vi "Header Footer Modify Image Cell.vi"(2 "Header or Footer":T1, 5 "Modify Image Cell":bool, 9 "Header or Footer Complete Cluster IN":T2, 11 "error in (no error)":errorcluster) -> (10 "Header or Footer Complete Cluster OUT":T2, 15 "error out":errorcluster)   [LabVIEW 2013]
doc: "Version 1.0\nDeveloped by Jean-Marc Simard\nCopyright © 2010, Exaprom Inc.\nAll rights reserved.\nLicense: BSD\n\nWith iTextSharp 4.1.6 (http://itextsharp.sourceforge.net)\nunder Mozilla Public License Version 1.1\n(http://www.mozilla.org/MPL/MPL-1.1.html)"
uses:
  Controls/Header Footer Complete Cluster.ctl
  Controls/Header Footer Cluster with references.ctl
  Controls/Header Footer Type.ctl
  Controls/Header footer horiz alignment.ctl
  Controls/Cell Vertical alignment.ctl
  Controls/Page number.ctl
  C:/Users/MaxCorp/Documents/GitHub/TopView/DLL/itextsharp.dll
  DLL/itextsharp.dll
  Controls/Font cluster.ctl
  Controls/Font size.ctl
  Controls/Font color.ctl
  Controls/Header Footer Line.ctl
  Controls/Header or Footer.ctl
panel:
  # "X"
  # "Y"
  # "X"
  # "Y"
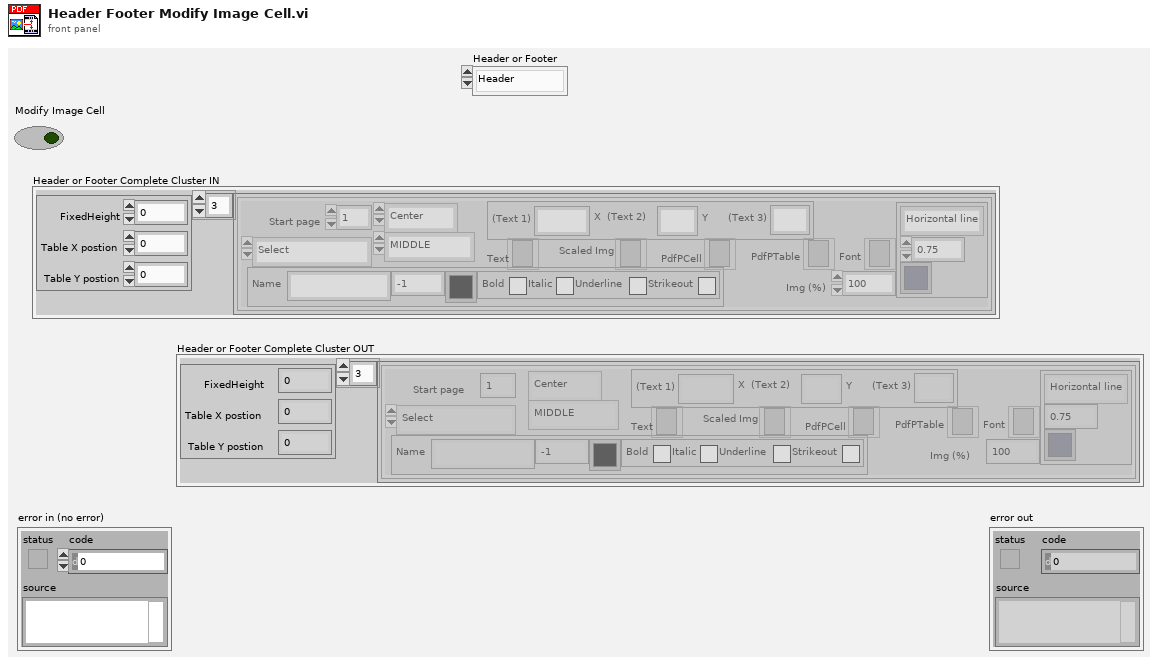
[diagram p1: front panel]
types:
  T1 = typedef "Header or Footer.ctl" = enum16{"Header", "Footer"}
  T2 = typedef "Header Footer Complete Cluster.ctl" = cluster{"Table position":cluster{"FixedHeight":dbl, "Table X postion":dbl, "Table Y postion":dbl}, "Header Footer Cluster with references [ ]":T3[]}
  T3 = typedef "Header Footer Cluster with references.ctl" = cluster{"Start page":i32, "Type":T4, "Alignment":T5, "Vertical Alignement":T6, "Page #":T7, "Text":refnum<k24>, "Scaled Img":refnum<k24>, "PdfPCell":refnum<k24>, "PdfPTable":refnum<k24>, "Font Cluster":T8, "Font ":refnum<k24>, "Img (%)":sgl, "Line":cluster{"Line":T11, "Thickness (points)":sgl, "Colour":T10}}
  T4 = typedef "Header Footer Type.ctl" = enum16{"Select", "Text", "Text + hyperlink", "Page number", "Image", "Image + hyperlink"}
  T5 = typedef "Header footer horiz alignment.ctl" = enum16{"Left", "Center", "Right"}
  T6 = typedef "Cell Vertical alignment.ctl" = enum16{"TOP", "MIDDLE", "BOTTOM"}
  T7 = typedef "Page number.ctl" = cluster{"Text 1":string, "Text 2":string, "Text 3":string}
  T8 = typedef "Font cluster.ctl" = cluster{"Name":string, "Size":T9, "Color":T10, "Style":cluster{"Bold":bool, "Italic":bool, "Underline":bool, "Strikeout":bool}}
  T9 = typedef "Font size.ctl" = sgl
  T10 = typedef "Font color.ctl" = u32
  T11 = typedef "Header Footer Line.ctl" = enum16{"No line", "Horizontal line"}
  T12 = cluster{"FixedHeight":dbl, "Table X postion":dbl, "Table Y postion":dbl}
  T13 = cluster{"Table position":cluster{"FixedHeight":dbl, "Table X postion":dbl, "Table Y postion":dbl}, "Header Footer Cluster with references [ ]":T3[]}
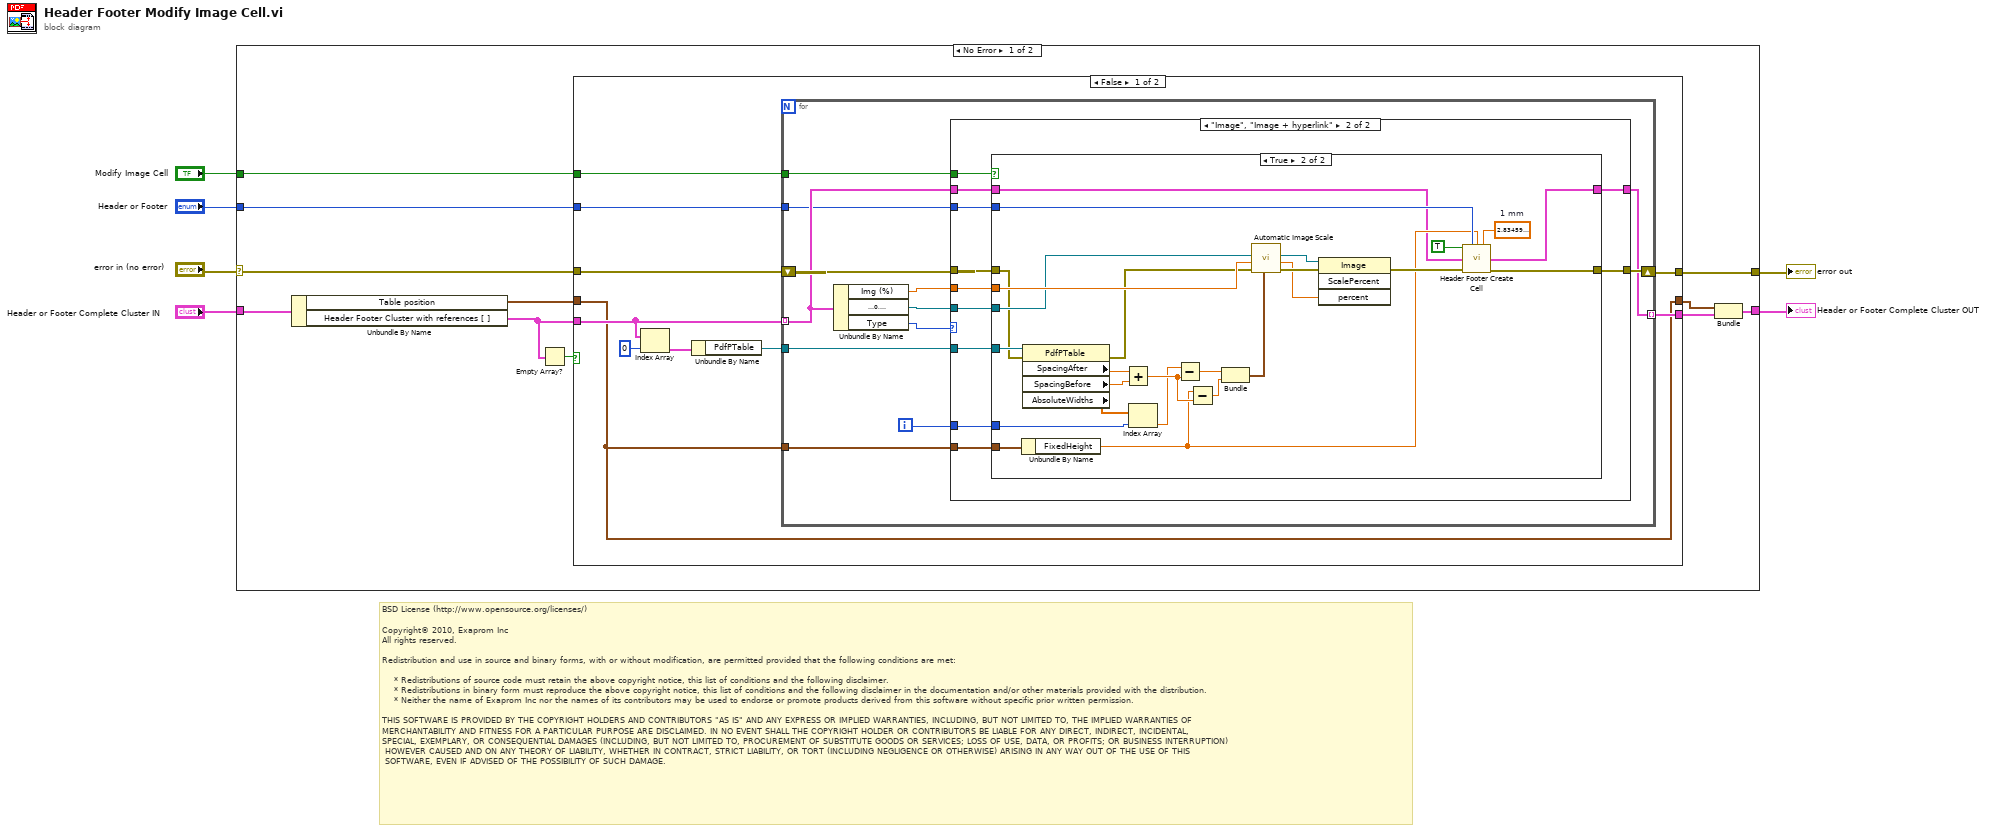
[diagram p0: block diagram]
diagram:
  # "BSD License (http://www.opensource.org/licenses/)\n\nCopyright© 2010, Exaprom Inc\nAll rights reserved.\n\nRedistribution and use in source and binary forms, with or without modification, are permitted provided that the following conditions are met:\n\n    * Redistributions of source code must retain the above copyright notice, this list of conditions and the following disclaimer.\n    * Redistributions in binary form must reproduce the above copyright notice, this list of conditions and the following disclaimer in the documentation and/or other materials provided with the distribution.\n    * Neither the name of Exaprom Inc nor the names of its contributors may be used to endorse or promote products derived from this software without specific prior written permission.\n\nTHIS SOFTWARE IS PROVIDED BY THE COPYRIGHT HOLDERS AND CONTRIBUTORS \"AS IS\" AND ANY EXPRESS OR IMPLIED WARRANTIES, INCLUDING, BUT NOT LIMITED TO, THE IMPLIED WARRANTIES OF \nMERCHANTABILITY AND FITNESS FOR A PARTICULAR PURPOSE ARE DISCLAIMED. IN NO EVENT SHALL THE COPYRIGHT HOLDER OR CONTRIBUTORS BE LIABLE FOR ANY DIRECT, INDIRECT, INCIDENTAL,\nSPECIAL, EXEMPLARY, OR CONSEQUENTIAL DAMAGES (INCLUDING, BUT NOT LIMITED TO, PROCUREMENT OF SUBSTITUTE GOODS OR SERVICES; LOSS OF USE, DATA, OR PROFITS; OR BUSINESS INTERRUPTION)\n HOWEVER CAUSED AND ON ANY THEORY OF LIABILITY, WHETHER IN CONTRACT, STRICT LIABILITY, OR TORT (INCLUDING NEGLIGENCE OR OTHERWISE) ARISING IN ANY WAY OUT OF THE USE OF THIS\n SOFTWARE, EVEN IF ADVISED OF THE POSSIBILITY OF SUCH DAMAGE."
  n1 = case shown="No Error" "error in (no error)" {
    selector: "error in (no error)" -> [w16 w85]
    tunnel: "Header or Footer Complete Cluster IN" -> [w15 w84]
    tunnel: [w17 w85] -> w6
    tunnel: [w14 w84] -> w2
    tunnel: "Header or Footer" -> [w13 _]
    tunnel: "Modify Image Cell" -> [w10 _]
    frame No Error {
      n2 = Unbundle By Name(w15) -> ("Table position"=w11:T12, "Header Footer Cluster with references [ ]"=w7:T3[])
      n3 = Empty Array?(array=w7) -> (empty?=w8:bool)
      n4 = case shown="False" w8 {
        tunnel: [w27 w83] -> w17
        tunnel: w16 -> [w26 w83]
        tunnel: w7 -> [w22 w82]
        tunnel: w13 -> [w21 _]
        tunnel: [w20 w82] -> w12
        tunnel: w11 -> [w18 w81]
        tunnel: w10 -> [w19 _]
        tunnel: [w18 w81] -> w9
        frame False {
          n5 = Index Array(array=w22, index=0) -> (element=w24:T3)
          n6 = Unbundle By Name(w24) -> ("PdfPTable"=w23:refnum<k24>)
          n7 = for {
            tunnel: w22 -> [w32] mode=indexing
            tunnel: w23 -> [w35]
            tunnel: w18 -> [w37]
            shift-right: [w30] -> w27
            shift-left: w26 -> [w38]
            tunnel: w21 -> [w31]
            tunnel: [w29] -> w20 mode=indexing
            tunnel: w19 -> [w28]
            i -> [w36]
            n8 = Unbundle By Name(w32) -> ("Img (%)"=w33:sgl, "Scaled Img"=w34:refnum<k24>, "Type"=w39:T4)
            n9 = case shown="\"Image\", \"Image + hyperlink\"" w39 {
              tunnel: w38 -> [w40 w52]
              tunnel: [w40 w51] -> w30
              tunnel: w35 -> [_ w50]
              tunnel: w36 -> [_ w49]
              tunnel: w37 -> [_ w48]
              tunnel: w34 -> [_ w47]
              tunnel: w33 -> [_ w46]
              tunnel: w32 -> [w41 w45]
              tunnel: w31 -> [_ w44]
              tunnel: [w41 w43] -> w29
              tunnel: w28 -> [_ w42]
              frame "Text", Default {
              }
              frame "Image", "Image + hyperlink" {
                n10 = case shown="True" w42 {
                  tunnel: w46 -> [_ w78]
                  tunnel: w52 -> [w54 w64]
                  tunnel: [w54 w61] -> w51
                  tunnel: w50 -> [_ w76]
                  tunnel: w49 -> [_ w75]
                  tunnel: w48 -> [_ w67]
                  tunnel: w47 -> [_ w65]
                  tunnel: w45 -> [w53 w56]
                  tunnel: w44 -> [_ w59]
                  tunnel: [w53 w55] -> w43
                  frame False {
                  }
                  frame True {
                    w60 = sgl 2.8346  # 1 mm
                    n11 = Unbundle By Name(w67) -> ("FixedHeight"=w58:dbl)
                    n12 = property class="PdfPTable"(reference=w76, error in=w64) -> (error out=w63:errorcluster, "SpacingAfter"=w71:sgl, "SpacingBefore"=w70:sgl, "AbsoluteWidths"=w74:sgl[])  [unwired: 1 out]
                    n13 = Add(x=w71, y=w70) -> (x+y=w69:sgl)
                    n14 = Index Array(array=w74, index=w75) -> (element=w68:sgl)
                    n15 = Subtract(x=w68, y=w69) -> (x-y=w73:sgl)
                    n16 = Subtract(x=w58, y=w69) -> (x-y=w72:dbl)
                    n17 = Bundle(w73, w72) -> (w66:cluster{sgl, dbl})  [unwired: 1 out]
                    n18 = call "Automatic Image Scale.vi"("Box"=w66, "error in (no error)"=w63, "Scale percent IN"=w78, "GetInstanceImage IN"=w65) -> ("error out"=w80:errorcluster, "Scale percent OUT"=w77:sgl, "GetInstanceImage OUT"=w79:refnum<k24>)  [unwired: 2 in, 3 out]
                    n19 = invoke class="Image" method="ScalePercent"(reference=w79, error in=w80, "percent"=w77) -> (error out=w62:errorcluster)  [unwired: 1 in, 3 out]
                    n20 = call "Header Footer Create Cell.vi"("Change format?"=TRUE, "Header or Footer"=w59, "FixedHeight (points)"=w58, "Padding (points)"=w60, "Header Footer Cluster with references IN"=w56, "error in (no error)"=w62) -> ("Header Footer Cluster with references OUT"=w55:T3, "error out"=w61:errorcluster)  [unwired: 2 in, 6 out]
                  }
                }
              }
            }
          }
        }
        frame True {
        }
      }
      n21 = Bundle("Table position"=w9, "Header Footer Cluster with references [ ]"=w12) -> (w14:T13)  [unwired: 1 out]
    }
    frame Error {
    }
  }
  "error out" <- w6
  "Header or Footer Complete Cluster OUT" <- w2
